vi "Func-엑셀 데이터를 그래프로 출력.vi"() -> ()   [LabVIEW 2015] (continued)
2.92\t19.328\n4.167\t2.85\t19.245\n4.083\t2.77\t19.179\n4\t2.68\t19.098\n3.917\t2.61\t19.025\n3.833\t2.53\t18.952\n3.75\t2.46\t18.87\n3.667\t2.38\t18.793\n3.583\t2.29\t18.723\n3.5\t2.22\t18.654\n3.417\t2.11\t18.582\n3.333\t2.03\t18.503\n3.25\t1.96\t18.435\n3.3\t1.89\t18.371\n3.3\t1.89\t18.367\n3.3\t1.88\t18.361\n3.3\t1.87\t18.354\n3.3\t1.86\t18.349\n3.3\t1.85\t18.337\n3.3\t1.85\t18.327\n3.3\t1.85\t18.316\n3.3\t1.84\t18.306\n3.3\t1.83\t18.299\n3.3\t1.83\t18.291\n3.3\t1.82\t18.284\n3.3\t1.81\t18.278\n3.3\t1.8\t18.274\n3.3\t1.79\t18.265\n3.3\t1.77\t18.259\n3.3\t1.77\t18.254\n3.3\t1.77\t18.244\n3.3\t1.75\t18.235\n3.3\t1.76\t18.228\n3.3\t1.74\t18.222\n3.3\t1.74\t18.214\n3.3\t1.72\t18.208\n3.3\t1.72\t18.2\n3.3\t1.7\t18.195\n3.3\t1.7\t18.186\n3.3\t1.69\t18.171\n3.3\t1.69\t18.166\n3.3\t1.69\t18.153\n3.3\t1.69\t18.148\n3.3\t1.68\t18.142\n3.3\t1.66\t18.139\n3.3\t1.65\t18.134\n3.3\t1.64\t18.131\n3.3\t1.64\t18.121\n3.3\t1.64\t18.115\n3.3\t1.63\t18.108\n3.3\t1.62\t18.097\n3.3\t1.62\t18.088\n3.3\t1.61\t18.081\n3.3\t1.61\t18.074\n3.3\t1.6\t18.065\n3.3\t1.6\t18.056\n3.3\t1.6\t18.046\n3.3\t1.59\t18.039\n3.3\t1.58\t18.031\n3.3\t1.58\t18.023\n3.3\t1.57\t18.019\n3.3\t1.57\t18.013\n3.3\t1.56\t18.006\n3.3\t1.55\t17.999\n3.3\t1.54\t17.993\n3.3\t1.53\t17.982\n3.3\t1.52\t17.974\n3.3\t1.52\t17.968\n3.3\t1.52\t17.958\n3.3\t1.52\t17.952\n3.3\t1.52\t17.945\n3.3\t1.52\t17.937\n3.3\t1.52\t17.93\n3.3\t1.51\t17.927\n3.3\t1.51\t17.919\n3.3\t1.5\t17.912\n3.3\t1.49\t17.907\n3.3\t1.49\t17.897\n3.3\t1.49\t17.892\n3.3\t1.48\t17.877\n3.3\t1.47\t17.871\n3.3\t1.48\t17.868\n3.3\t1.47\t17.86\n3.3\t1.46\t17.852\n3.3\t1.45\t17.846\n3.3\t1.45\t17.838\n3.3\t1.44\t17.832\n3.3\t1.43\t17.823\n3.3\t1.43\t17.814\n3.3\t1.43\t17.806\n3.3\t1.43\t17.8\n3.3\t1.42\t17.793\n3.3\t1.42\t17.788\n3.3\t1.41\t17.781\n3.3\t1.4\t17.771\n3.3\t1.4\t17.763\n3.3\t1.4\t17.755\n3.3\t1.4\t17.747\n3.3\t1.4\t17.74\n3.3\t1.4\t17.732\n3.3\t1.4\t17.725\n3.3\t1.4\t17.719\n3.3\t1.41\t17.709\n3.3\t1.4\t17.698\n3.3\t1.4\t17.689\n3.3\t1.39\t17.68\n3.3\t1.4\t17.672\n3.3\t1.39\t17.672\n3.3\t1.39\t17.668\n3.3\t1.39\t17.661\n3.3\t1.38\t17.658\n3.3\t1.39\t17.655\n3.3\t1.39\t17.643\n3.3\t1.39\t17.633\n3.3\t1.39\t17.627\n3.3\t1.4\t17.614\n3.3\t1.39\t17.607\n3.3\t1.4\t17.6\n3.3\t1.4\t17.593\n3.3\t1.4\t17.586\n3.3\t1.39\t17.579\n3.3\t1.39\t17.573\n3.3\t1.39\t17.565\n3.3\t1.39\t17.56\n3.3\t1.39\t17.554\n3.3\t1.39\t17.549\n3.3\t1.39\t17.545\n3.3\t1.39\t17.541\n3.3\t1.39\t17.533\n3.3\t1.39\t17.523\n3.3\t1.39\t17.509\n3.3\t1.4\t17.501\n3.3\t1.4\t17.493\n3.3\t1.41\t17.479\n3.3\t1.41\t17.474\n3.3\t1.4\t17.47\n3.3\t1.4\t17.466\n3.3\t1.4\t17.461\n3.3\t1.39\t17.452\n3.3\t1.4\t17.442\n3.3\t1.41\t17.435\n3.3\t1.4\t17.426\n3.3\t1.4\t17.416\n3.3\t1.41\t17.406\n3.3\t1.41\t17.4\n3.3\t1.41\t17.391\n3.3\t1.43\t17.386\n3.3\t1.43\t17.38\n3.3\t1.43\t17.37\n3.3\t1.43\t17.364\n3.3\t1.43\t17.356\n3.3\t1.43\t17.35\n3.3\t1.43\t17.34\n3.3\t1.43\t17.332\n3.3\t1.43\t17.321\n3.3\t1.43\t17.31\n3.3\t1.43\t17.303\n3.3\t1.43\t17.296\n3.3\t1.44\t17.29\n3.3\t1.44\t17.282\n3.3\t1.45\t17.275\n3.3\t1.45\t17.272\n3.3\t1.45\t17.268\n3.3\t1.46\t17.258\n3.3\t1.45\t17.252\n3.3\t1.46\t17.248\n3.3\t1.45\t17.236\n3.3\t1.47\t17.231\n3.3\t1.47\t17.225\n3.3\t1.48\t17.215\n3.3\t1.48\t17.21\n3.3\t1.49\t17.204\n3.3\t1.49\t17.199\n3.3\t1.48\t17.193\n3.3\t1.48\t17.185\n3.3\t1.49\t17.175\n3.3\t1.49\t17.168\n3.3\t1.5\t17.159\n3.3\t1.5\t17.152\n3.3\t1.5\t17.143\n3.3\t1.5\t17.135\n3.3\t1.51\t17.13\n3.3\t1.52\t17.121\n3.3\t1.52\t17.118\n3.3\t1.52\t17.109\n3.3\t1.53\t17.104\n3.3\t1.53\t17.099\n3.3\t1.53\t17.089\n3.3\t1.53\t17.083\n3.3\t1.53\t17.075\n3.3\t1.53\t17.07\n3.3\t1.54\t17.059\n3.3\t1.55\t17.051\n3.3\t1.55\t17.043\n3.3\t1.56\t17.036\n3.3\t1.57\t17.03\n3.3\t1.57\t17.018\n3.3\t1.57\t17.013\n3.3\t1.58\t17.009\n3.3\t1.58\t16.999\n3.3\t1.59\t16.991\n3.3\t1.6\t16.981\n3.3\t1.6\t16.971\n3.3\t1.61\t16.965\n3.3\t1.62\t16.955\n3.3\t1.62\t16.95\n3.3\t1.62\t16.95\n3.3\t1.62\t16.946\n3.3\t1.63\t16.938\n3.3\t1.64\t16.932\n3.3\t1.64\t16.921\n3.3\t1.65\t16.913\n3.3\t1.66\t16.902\n3.3\t1.66\t16.893\n3.3\t1.66\t16.888\n3.3\t1.67\t16.88\n3.3\t1.68\t16.875\n3.3\t1.69\t16.87\n3.3\t1.69\t16.867\n3.3\t1.69\t16.86\n3.3\t1.69\t16.854\n3.3\t1.7\t16.851\n3.3\t1.71\t16.843\n3.3\t1.72\t16.836\n3.3\t1.73\t16.828\n3.3\t1.74\t16.817\n3.3\t1.75\t16.81\n3.3\t1.75\t16.8\n3.3\t1.75\t16.791\n3.3\t1.76\t16.782\n3.3\t1.76\t16.772\n3.3\t1.76\t16.763\n3.3\t1.77\t16.757\n3.3\t1.77\t16.753\n3.3\t1.78\t16.745\n3.3\t1.78\t16.737\n3.3\t1.79\t16.734\n3.3\t1.8\t16.729\n3.3\t1.81\t16.72\n3.3\t1.81\t16.711\n3.3\t1.82\t16.702\n3.3\t1.83\t16.698\n3.3\t1.83\t16.688\n3.3\t1.84\t16.677\n3.3\t1.85\t16.675\n3.3\t1.85\t16.672\n3.3\t1.85\t16.663\n3.3\t1.86\t16.657\n3.3\t1.86\t16.653\n3.3\t1.87\t16.646\n3.3\t1.88\t16.637\n3.3\t1.89\t16.63\n3.3\t1.9\t16.625\n3.3\t1.91\t16.62\n3.3\t1.91\t16.617\n3.3\t1.92\t16.608\n3.3\t1.93\t16.604\n3.3\t1.94\t16.597\n3.3\t1.94\t16.584\n3.3\t1.94\t16.574\n3.3\t1.95\t16.569\n3.3\t1.95\t16.562\n3.3\t1.95\t16.55\n3.3\t1.96\t16.543\n3.3\t1.97\t16.536\n3.3\t1.98\t16.532\n3.3\t1.99\t16.524\n3.3\t2\t16.511\n3.3\t2.01\t16.507\n3.3\t2.02\t16.502\n3.3\t2.02\t16.493\n3.3\t2.03\t16.491\n3.3\t2.03\t16.483\n3.3\t2.04\t16.482\n3.3\t2.05\t16.478\n3.3\t2.05\t16.475\n3.3\t2.06\t16.468\n3.3\t2.07\t16.46\n3.3\t2.07\t16.451\n3.3\t2.07\t16.441\n3.3\t2.08\t16.435\n3.3\t2.09\t16.424\n3.3\t2.09\t16.416\n3.3\t2.1\t16.41\n3.3\t2.1\t16.4\n3.3\t2.11\t16.392\n3.3\t2.11\t16.385\n3.3\t2.12\t16.38\n3.3\t2.13\t16.376\n3.3\t2.14\t16.369\n3.3\t2.14\t16.36\n3.3\t2.15\t16.357\n3.3\t2.16\t16.351\n3.3\t2.17\t16.343\n3.3\t2.17\t16.336\n3.3\t2.18\t16.333\n3.3\t2.19\t16.334\n3.3\t2.19\t16.327\n3.3\t2.19\t16.32\n3.3\t2.2\t16.307\n3.3\t2.21\t16.298\n3.3\t2.22\t16.287\n3.3\t2.23\t16.274\n3.3\t2.24\t16.27\n3.3\t2.25\t16.265\n3.3\t2.25\t16.263\n3.3\t2.25\t16.262\n3.3\t2.25\t16.257\n3.3\t2.26\t16.251\n3.3\t2.27\t16.244\n3.3\t2.27\t16.236\n3.3\t2.28\t16.225\n3.3\t2.29\t16.218\n3.3\t2.3\t16.212\n3.3\t2.3\t16.204\n3.3\t2.31\t16.196\n3.3\t2.31\t16.195\n3.3\t2.32\t16.186\n3.3\t2.32\t16.179\n3.3\t2.33\t16.176\n3.3\t2.34\t16.169\n3.3\t2.35\t16.164\n3.3\t2.36\t16.155\n3.3\t2.36\t16.15\n3.3\t2.36\t16.145\n3.3\t2.36\t16.136\n3.3\t2.37\t16.127\n3.3\t2.37\t16.12\n3.3\t2.38\t16.112\n3.3\t2.39\t16.102\n3.3\t2.39\t16.096\n3.3\t2.4\t16.092\n3.3\t2.4\t16.085\n3.3\t2.4\t16.079\n3.3\t2.41\t16.074\n3.3\t2.42\t16.066\n3.3\t2.43\t16.06\n3.3\t2.44\t16.054\n3.3\t2.44\t16.044\n3.3\t2.44\t16.041\n3.3\t2.45\t16.038\n3.3\t2.45\t16.028\n3.3\t2.45\t16.022\n3.3\t2.46\t16.014\n3.3\t2.47\t16.007\n3.3\t2.48\t15.999\n3.3\t2.49\t15.994\n3.3\t2.5\t15.99\n3.3\t2.51\t15.984\n3.3\t2.51\t15.98\n3.3\t2.51\t15.973\n3.3\t2.52\t15.966\n3.3\t2.52\t15.96\n3.3\t2.52\t15.95\n3.3\t2.52\t15.945\n3.3\t2.52\t15.939\n3.3\t2.53\t15.93\n3.3\t2.53\t15.926\n3.3\t2.55\t15.92\n3.3\t2.55\t15.917\n3.3\t2.57\t15.909\n3.3\t2.57\t15.897\n3.3\t2.58\t15.894\n3.3\t2.58\t15.891\n3.3\t2.59\t15.884\n3.3\t2.6\t15.874\n3.3\t2.6\t15.871\n3.3\t2.61\t15.866\n3.3\t2.61\t15.859\n3.3\t2.61\t15.852\n3.3\t2.62\t15.848\n3.3\t2.63\t15.844\n3.3\t2.63\t15.841\n3.3\t2.63\t15.834\n3.3\t2.64\t15.831\n3.3\t2.65\t15.822\n3.3\t2.66\t15.812\n3.3\t2.66\t15.806\n3.3\t2.68\t15.799\n3.3\t2.68\t15.793\n3.3\t2.69\t15.786\n3.3\t2.69\t15.782\n3.3\t2.69\t15.774\n3.3\t2.69\t15.771\n3.3\t2.69\t15.762\n3.3\t2.69\t15.754\n3.3\t2.7\t15.748\n3.3\t2.71\t15.74\n3.3\t2.72\t15.732\n3.3\t2.73\t15.724\n3.3\t2.74\t15.721\n3.3\t2.74\t15.714\n3.3\t2.74\t15.709\n3.3\t2.75\t15.71\n3.3\t2.76\t15.703\n3.3\t2.77\t15.701\n3.3\t2.78\t15.697\n3.3\t2.78\t15.689\n3.3\t2.79\t15.684\n3.3\t2.79\t15.676\n3.3\t2.79\t15.666\n3.3\t2.8\t15.66\n3.3\t2.81\t15.652\n3.3\t2.82\t15.644\n3.3\t2.83\t15.637\n3.3\t2.84\t15.63\n3.3\t2.84\t15.624\n3.3\t2.84\t15.617\n3.3\t2.84\t15.614\n3.3\t2.84\t15.605\n3.3\t2.85\t15.603\n3.3\t2.86\t15.599\n3.3\t2.87\t15.592\n3.3\t2.87\t15.588\n3.3\t2.88\t15.582\n3.3\t2.88\t15.579\n3.3\t2.88\t15.572\n3.3\t2.88\t15.566\n3.3\t2.89\t15.563\n3.3\t2.89\t15.557\n3.3\t2.9\t15.552\n3.3\t2.91\t15.543\n3.3\t2.93\t15.536\n3.3\t2.92\t15.533\n3.3\t2.93\t15.523\n3.3\t2.93\t15.52\n3.3\t2.93\t15.514\n3.3\t2.93\t15.509\n3.3\t2.94\t15.507\n3.3\t2.94\t15.503\n3.3\t2.95\t15.497\n3.3\t2.95\t15.493\n3.3\t2.96\t15.488\n3.3\t2.97\t15.481\n3.3\t2.98\t15.473\n3.3\t2.98\t15.464\n3.3\t2.98\t15.455\n3.3\t2.99\t15.448\n3.3\t2.99\t15.447\n3.3\t2.99\t15.441\n3.3\t3\t15.435\n3.3\t3.01\t15.43\n3.3\t3.01\t15.425\n3.3\t3.01\t15.421\n3.3\t3.02\t15.414\n3.3\t3.02\t15.407\n3.3\t3.02\t15.404\n3.3\t3.02\t15.395\n3.3\t3.03\t15.391\n3.3\t3.03\t15.389\n3.3\t3.03\t15.382\n3.3\t3.03\t15.378\n3.3\t3.04\t15.373\n3.3\t3.04\t15.369\n3.3\t3.05\t15.363\n3.3\t3.05\t15.354\n3.3\t3.05\t15.346\n3.3\t3.05\t15.337\n3.3\t3.06\t15.335\n3.3\t3.07\t15.329\n3.3\t3.07\t15.328\n3.3\t3.08\t15.325\n3.3\t3.08\t15.319\n3.3\t3.08\t15.314\n3.3\t3.09\t15.307\n3.3\t3.09\t15.299\n3.3\t3.1\t15.291\n3.3\t3.1\t15.286\n3.3\t3.11\t15.283\n3.3\t3.11\t15.278\n3.3\t3.11\t15.272\n3.3\t3.11\t15.267\n3.3\t3.11\t15.264\n3.3\t3.11\t15.26\n3.3\t3.11\t15.252\n3.3\t3.11\t15.248\n3.3\t3.12\t15.248\n3.3\t3.13\t15.238\n3.3\t3.13\t15.232\n3.3\t3.13\t15.224\n3.3\t3.13\t15.216\n3.3\t3.14\t15.212\n3.3\t3.14\t15.208\n3.3\t3.14\t15.204\n3.3\t3.15\t15.199\n3.3\t3.15\t15.198\n3.3\t3.16\t15.195\n3.3\t3.16\t15.19\n3.3\t3.17\t15.187\n3.3\t3.17\t15.18\n3.3\t3.18\t15.175\n3.3\t3.18\t15.168\n3.3\t3.19\t15.163\n3.3\t3.19\t15.154\n3.3\t3.19\t15.146\n3.3\t3.19\t15.145\n3.3\t3.19\t15.142\n3.3\t3.19\t15.139\n3.3\t3.2\t15.131\n3.3\t3.2\t15.128\n3.3\t3.2\t15.123\n3.3\t3.2\t15.115\n3.3\t3.2\t15.112\n3.3\t3.21\t15.107\n3.3\t3.22\t15.103\n3.3\t3.22\t15.102\n3.3\t3.22\t15.096\n3.3\t3.23\t15.091\n3.3\t3.23\t15.084\n3.3\t3.23\t15.077\n3.3\t3.24\t15.07\n3.3\t3.25\t15.066\n3.3\t3.25\t15.063\n3.3\t3.24\t15.055\n3.3\t3.24\t15.049\n3.3\t3.25\t15.048\n3.3\t3.25\t15.042\n3.3\t3.25\t15.037\n3.3\t3.26\t15.031\n3.3\t3.26\t15.03\n3.3\t3.25\t15.028\n3.3\t3.25\t15.025\n3.3\t3.25\t15.021\n3.3\t3.26\t15.02\n3.3\t3.27\t15.016\n3.3\t3.28\t15.006\n3.3\t3.3\t15.001\n3.3\t3.3\t14.996\n3.3\t3.3\t14.988\n3.3\t3.3\t14.981\n3.3\t3.3\t14.979\n3.3\t3.3\t14.974\n3.3\t3.3\t14.969\n3.3\t3.3\t14.964\n3.3\t3.3\t14.961\n3.3\t3.3\t14.959\n3.3\t3.3\t14.952\n3.3\t3.3\t14.95\n3.3\t3.3\t14.948\n3.3\t3.3\t14.946\n3.3\t3.3\t14.94\n3.3\t3.3\t14.933\n3.3\t3.3\t14.931\n3.3\t3.3\t14.925\n3.3\t3.3\t14.92\n3.3\t3.3\t14.912\n3.3\t3.3\t14.9\n3.3\t3.3\t14.895\n3.3\t3.3\t14.889\n3.3\t3.3\t14.88\n3.3\t3.3\t14.873\n3.3\t3.3\t14.867\n3.3\t3.3\t14.866\n3.3\t3.3\t14.864\n3.3\t3.3\t14.862\n3.3\t3.3\t14.855\n3.3\t3.3\t14.855\n3.3\t3.3\t14.855\n3.3\t3.3\t14.848\n3.3\t3.3\t14.843\n3.3\t3.3\t14.84\n3.3\t3.3\t14.837\n3.3\t3.3\t14.836\n3.3\t3.3\t14.833\n3.3\t3.3\t14.83\n3.3\t3.3\t14.827\n3.3\t3.3\t14.823\n3.3\t3.3\t14.817\n3.3\t3.3\t14.813\n3.3\t3.31\t14.81\n3.3\t3.31\t14.805\n3.3\t3.31\t14.8\n3.3\t3.31\t14.798\n3.3\t3.31\t14.79\n3.3\t3.31\t14.787\n3.3\t3.31\t14.782\n3.3\t3.31\t14.778\n3.3\t3.31\t14.777\n3.3\t3.31\t14.77\n3.3\t3.31\t14.765\n3.3\t3.31\t14.758\n3.3\t3.31\t14.752\n3.3\t3.31\t14.743\n3.3\t3.31\t14.736\n3.3\t3.31\t14.734\n3.3\t3.31\t14.733\n3.3\t3.31\t14.727\n3.3\t3.31\t14.721\n3.3\t3.31\t14.715\n3.3\t3.31\t14.71\n3.3\t3.31\t14.708\n3.3\t3.31\t14.701\n3.3\t3.31\t14.698\n3.3\t3.31\t14.7\n3.3\t3.31\t14.7\n3.3\t3.31\t14.696\n3.3\t3.31\t14.691\n3.3\t3.31\t14.686\n3.3\t3.31\t14.684\n3.3\t3.31\t14.679\n3.3\t3.31\t14.673\n3.3\t3.31\t14.671\n3.3\t3.31\t14.667\n3.3\t3.31\t14.663\n3.3\t3.31\t14.659\n3.3\t3.31\t14.658\n3.3\t3.32\t14.653\n3.3\t3.32\t14.648\n3.3\t3.32\t14.644\n3.3\t3.32\t14.638\n3.3\t3.32\t14.63\n3.3\t3.32\t14.624\n3.3\t3.32\t14.62\n3.3\t3.32\t14.618\n3.3\t3.32\t14.616\n3.3\t3.32\t14.613\n3.3\t3.32\t14.609\n3.3\t3.32\t14.608\n3.3\t3.32\t14.603\n3.3\t3.32\t14.596\n3.3\t3.32\t14.591\n3.3\t3.32\t14.586\n3.3\t3.32\t14.585\n3.3\t3.32\t14.577\n3.3\t3.32\t14.575\n3.3\t3.32\t14.575\n3.3\t3.32\t14.567\n3.3\t3.32\t14.566\n3.3\t3.32\t14.561\n3.3\t3.32\t14.557\n3.3\t3.32\t14.55\n3.3\t3.32\t14.549\n3.3\t3.32\t14.55\n3.3\t3.32\t14.547\n3.3\t3.32\t14.546\n3.3\t3.32\t14.543\n3.3\t3.32\t14.541\n3.3\t3.32\t14.535\n3.3\t3.32\t14.526\n3.3\t3.32\t14.521\n3.3\t3.32\t14.513\n3.3\t3.32\t14.512\n3.3\t3.32\t14.511\n3.3\t3.32\t14.507\n3.3\t3.32\t14.507\n3.3\t3.32\t14.504\n3.3\t3.32\t14.505\n3.3\t3.32\t14.5\n3.3\t3.32\t14.496\n3.3\t3.32\t14.495\n3.3\t3.32\t14.491\n3.3\t3.32\t14.489\n3.3\t3.32\t14.486\n3.3\t3.32\t14.479\n3.3\t3.32\t14.477\n3.3\t3.32\t14.47\n3.3\t3.32\t14.467\n3.3\t3.32\t14.462\n3.3\t3.32\t14.457\n3.3\t3.32\t14.454\n3.3\t3.32\t14.449\n3.3\t3.32\t14.448\n3.3\t3.32\t14.44\n3.3\t3.32\t14.439\n3.3\t3.32\t14.435\n3.3\t3.32\t14.426\n3.3\t3.32\t14.421\n3.3\t3.32\t14.418\n3.3\t3.32\t14.412\n3.3\t3.32\t14.407\n3.3\t3.32\t14.407\n3.3\t3.32\t14.408\n3.3\t3.32\t14.41\n3.3\t3.32\t14.407\n3.3\t3.32\t14.407\n3.3\t3.32\t14.404\n3.3\t3.32\t14.396\n3.3\t3.32\t14.388\n3.3\t3.32\t14.387\n3.3\t3.32\t14.387\n3.3\t3.32\t14.383\n3.3\t3.32\t14.381\n3.3\t3.32\t14.382\n3.3\t3.32\t14.377\n3.3\t3.32\t14.367\n3.3\t3.32\t14.359\n3.3\t3.32\t14.349\n3.3\t3.32\t14.345\n3.3\t3.33\t14.343\n3.3\t3.32\t14.342\n3.3\t3.33\t14.34\n3.3\t3.33\t14.336\n3.3\t3.33\t14.332\n3.3\t3.32\t14.332\n3.3\t3.32\t14.329\n3.3\t3.32\t14.322\n3.3\t3.32\t14.319\n3.3\t3.32\t14.32\n3.3\t3.33\t14.318\n3.3\t3.33\t14.313\n3.3\t3.33\t14.311\n3.3\t3.33\t14.311\n3.3\t3.33\t14.31\n3.3\t3.33\t14.306\n3.3\t3.32\t14.303\n3.3\t3.32\t14.301\n3.3\t3.32\t14.295\n3.3\t3.32\t14.291\n3.3\t3.33\t14.288\n3.3\t3.33\t14.284\n3.3\t3.33\t14.28\n3.3\t3.33\t14.275\n3.3\t3.33\t14.272\n3.3\t3.33\t14.268\n3.3\t3.33\t14.264\n3.3\t3.33\t14.264\n3.3\t3.33\t14.259\n3.3\t3.33\t14.257\n3.3\t3.33\t14.255\n3.3\t3.33\t14.252\n3.3\t3.33\t14.246\n3.3\t3.33\t14.241\n3.3\t3.33\t14.237\n3.3\t3.33\t14.233\n3.3\t3.33\t14.231\n3.3\t3.32\t14.223\n3.3\t3.32\t14.225\n3.3\t3.32\t14.223\n3.3\t3.32\t14.222\n3.3\t3.32\t14.22\n3.3\t3.32\t14.216\n3.3\t3.32\t14.216\n3.3\t3.33\t14.212\n3.3\t3.33\t14.208\n3.3\t3.33\t14.203\n3.3\t3.33\t14.196\n3.3\t3.32\t14.193\n3.3\t3.32\t14.191\n3.3\t3.32\t14.188\n3.3\t3.32\t14.183\n3.3\t3.32\t14.181\n3.3\t3.32\t14.182\n3.3\t3.32\t14.184\n3.3\t3.32\t14.181\n3.3\t3.32\t14.176\n3.3\t3.32\t14.179\n3.3\t3.32\t14.175\n3.3\t3.32\t14.173\n3.3\t3.32\t14.166\n3.3\t3.32\t14.159\n3.3\t3.32\t14.157\n3.3\t3.32\t14.153\n3.3\t3.32\t14.154\n3.3\t3.32\t14.152\n3.3\t3.32\t14.15\n3.3\t3.32\t14.15\n3.3\t3.32\t14.148\n3.3\t3.32\t14.145\n3.3\t3.32\t14.134\n3.3\t3.32\t14.131\n3.3\t3.32\t14.128\n3.3\t3.32\t14.123\n3.3\t3.32\t14.119\n3.3\t3.32\t14.118\n3.3\t3.32\t14.116\n3.3\t3.32\t14.11\n3.3\t3.32\t14.11\n3.3\t3.32\t14.104\n3.3\t3.32\t14.104\n3.3\t3.32\t14.098\n3.3\t3.32\t14.095\n3.3\t3.32\t14.099\n3.3\t3.32\t14.094\n3.3\t3.32\t14.091\n3.3\t3.32\t14.088\n3.3\t3.32\t14.087\n3.3\t3.32\t14.086\n3.3\t3.32\t14.079\n3.3\t3.32\t14.075\n3.3\t3.32\t14.07\n3.3\t3.32\t14.066\n3.3\t3.32\t14.064\n3.3\t3.32\t14.061\n3.3\t3.32\t14.059\n3.3\t3.32\t14.057\n3.3\t3.32\t14.056\n3.3\t3.32\t14.054\n3.3\t3.32\t14.05\n3.3\t3.32\t14.048\n3.3\t3.32\t14.044\n3.3\t3.32\t14.044\n3.3\t3.32\t14.039\n3.3\t3.32\t14.036\n3.3\t3.32\t14.031\n3.3\t3.32\t14.025\n3.3\t3.32\t14.025\n3.3\t3.32\t14.024\n3.3\t3.32\t14.019\n3.3\t3.32\t14.017\n3.3\t3.32\t14.02\n3.3\t3.32\t14.016\n3.3\t3.32\t14.013\n3.3\t3.32\t14.009\n3.3\t3.32\t14.01\n3.3\t3.32\t14.008\n3.3\t3.32\t14.004\n3.3\t3.32\t13.998\n3.3\t3.32\t13.994\n3.3\t3.32\t13.994\n3.3\t3.32\t13.986\n3.3\t3.32\t13.985\n3.3\t3.32\t13.979\n3.3\t3.32\t13.979\n3.3\t3.32\t13.979\n3.3\t3.32\t13.976\n3.3\t3.32\t13.973\n3.3\t3.32\t13.971\n3.3\t3.31\t13.969\n3.3\t3.31\t13.966\n3.3\t3.31\t13.962\n3.3\t3.31\t13.96\n3.3\t3.31\t13.959\n3.3\t3.31\t13.954\n3.3\t3.31\t13.951\n3.3\t3.31\t13.944\n3.3\t3.31\t13.943\n3.3\t3.31\t13.941\n3.3\t3.31\t13.939\n3.3\t3.31\t13.939\n3.3\t3.31\t13.939\n3.3\t3.31\t13.94\n3.3\t3.31\t13.936\n3.3\t3.31\t13.932\n3.3\t3.31\t13.927\n3.3\t3.31\t13.925\n3.3\t3.31\t13.92\n3.3\t3.31\t13.918\n3.3\t3.31\t13.914\n3.3\t3.31\t13.913\n3.3\t3.31\t13.91\n3.3\t3.31\t13.908\n3.3\t3.31\t13.905\n3.3\t3.31\t13.9\n3.3\t3.31\t13.898\n3.3\t3.31\t13.898\n3.3\t3.31\t13.893\n3.3\t3.31\t13.889\n3.3\t3.31\t13.889\n3.3\t3.31\t13.887\n3.3\t3.31\t13.886\n3.3\t3.31\t13.88\n3.3\t3.31\t13.878\n3.3\t3.31\t13.877\n3.3\t3.31\t13.875\n3.3\t3.31\t13.876\n3.3\t3.31\t13.871\n3.3\t3.31\t13.871\n3.3\t3.31\t13.869\n3.3\t3.31\t13.866\n3.3\t3.31\t13.865\n3.3\t3.31\t13.859\n3.3\t3.31\t13.863\n3.3\t3.31\t13.86\n3.3\t3.31\t13.858\n3.3\t3.31\t13.859\n3.3\t3.31\t13.854\n3.3\t3.31\t13.852\n3.3\t3.31\t13.845\n3.3\t3.31\t13.837\n3.3\t3.31\t13.837\n3.3\t3.31\t13.834\n3.3\t3.31\t13.831\n3.3\t3.31\t13.831\n3.3\t3.31\t13.831\n3.3\t3.31\t13.832\n3.3\t3.31\t13.827\n3.3\t3.31\t13.826\n3.3\t3.31\t13.82\n3.3\t3.31\t13.816\n3.3\t3.31\t13.813\n3.3\t3.31\t13.814\n3.3\t3.31\t13.812\n3.3\t3.31\t13.806\n3.3\t3.31\t13.807\n3.3\t3.31\t13.806\n3.3\t3.31\t13.804\n3.3\t3.31\t13.8\n3.3\t3.31\t13.799\n3.3\t3.31\t13.798\n3.3\t3.31\t13.796\n3.3\t3.3\t13.794\n3.3\t3.3\t13.795\n3.3\t3.3\t13.79\n3.3\t3.3\t13.787\n3.3\t3.31\t13.788\n3.3\t3.31\t13.788\n3.3\t3.31\t13.782\n3.3\t3.31\t13.778\n3.3\t3.31\t13.776\n3.3\t3.31\t13.773\n3.3\t3.31\t13.771\n3.3\t3.31\t13.769\n3.3\t3.31\t13.769\n3.3\t3.31\t13.767\n3.3\t3.31\t13.765\n3.3\t3.31\t13.764\n3.3\t3.31\t13.761\n3.3\t3.31\t13.755\n3.3\t3.31\t13.746\n3.3\t3.31\t13.745\n3.3\t3.31\t13.745\n3.3\t3.31\t13.739\n3.3\t3.31\t13.738\n3.3\t3.31\t13.74\n3.3\t3.31\t13.743\n3.3\t3.31\t13.739\n3.3\t3.31\t13.734\n3.3\t3.3\t13.732\n3.3\t3.3\t13.728\n3.3\t3.3\t13.726\n3.3\t3.3\t13.723\n3.3\t3.3\t13.723\n3.3\t3.3\t13.721\n3.3\t3.3\t13.714\n3.3\t3.3\t13.711\n3.3\t3.3\t13.709\n3.3\t3.3\t13.707\n3.3\t3.3\t13.705\n3.3\t3.3\t13.705\n3.3\t3.3\t13.706\n3.3\t3.3\t13.707\n3.3\t3.3\t13.702\n3.3\t3.3\t13.696\n3.3\t3.3\t13.693\n3.3\t3.3\t13.69\n3.3\t3.3\t13.687\n3.3\t3.3\t13.686\n3.3\t3.3\t13.687\n3.3\t3.3\t13.687\n3.3\t3.3\t13.686\n3.3\t3.3\t13.68\n3.3\t3.3\t13.678\n3.3\t3.3\t13.676\n3.3\t3.3\t13.673\n3.3\t3.3\t13.666\n3.3\t3.3\t13.666\n3.3\t3.3\t13.667\n3.3\t3.3\t13.666\n3.3\t3.3\t13.661\n3.3\t3.3\t13.657\n3.3\t3.3\t13.655\n3.3\t3.3\t13.655\n3.3\t3.3\t13.648\n3.3\t3.3\t13.645\n3.3\t3.3\t13.642\n3.3\t3.3\t13.641\n3.3\t3.3\t13.641\n3.3\t3.3\t13.641\n3.3\t3.3\t13.644\n3.3\t3.3\t13.641\n3.3\t3.3\t13.644\n3.3\t3.3\t13.639\n3.3\t3.3\t13.637\n3.3\t3.3\t13.635\n3.3\t3.3\t13.632\n3.3\t3.3\t13.63\n3.3\t3.3\t13.628\n3.3\t3.3\t13.628\n3.3\t3.3\t13.625\n3.3\t3.3\t13.623\n3.3\t3.3\t13.618\n3.3\t3.3\t13.618\n3.3\t3.3\t13.617\n3.3\t3.3\t13.612\n3.3\t3.3\t13.61\n3.3\t3.3\t13.608\n3.3\t3.3\t13.605\n3.3\t3.3\t13.603\n3.3\t3.3\t13.6\n3.3\t3.3\t13.599\n3.3\t3.3\t13.6\n3.3\t3.3\t13.598\n3.3\t3.3\t13.594\n3.3\t3.3\t13.591\n3.3\t3.3\t13.591\n3.3\t3.3\t13.589\n3.3\t3.3\t13.585\n3.3\t3.3\t13.582\n3.3\t3.3\t13.586\n3.3\t3.3\t13.586\n3.3\t3.3\t13.581\n3.3\t3.3\t13.576\n3.3\t3.3\t13.572\n3.3\t3.3\t13.57\n3.3\t3.3\t13.566\n3.3\t3.3\t13.561\n3.3\t3.3\t13.558\n3.3\t3.3\t13.557\n3.3\t3.3\t13.556\n3.3\t3.3\t13.557\n3.3\t3.3\t13.553\n3.3\t3.3\t13.552\n3.3\t3.3\t13.553\n3.3\t3.3\t13.549\n3.3\t3.3\t13.549\n3.3\t3.3\t13.548\n3.3\t3.3\t13.546\n3.3\t3.3\t13.545\n3.3\t3.3\t13.545\n3.3\t3.3\t13.545\n3.3\t3.3\t13.544\n3.3\t3.3\t13.539\n3.3\t3.3\t13.538\n3.3\t3.3\t13.534\n3.3\t3.3\t13.53\n3.3\t3.3\t13.529\n3.3\t3.3\t13.527\n3.3\t3.3\t13.526\n3.3\t3.3\t13.525\n3.3\t3.3\t13.527\n3.3\t3.3\t13.523\n3.3\t3.3\t13.517\n3.3\t3.3\t13.514\n3.3\t3.3\t13.512\n3.3\t3.3\t13.512\n3.3\t3.3\t13.508\n3.3\t3.3\t13.509\n3.3\t3.3\t13.51\n3.3\t3.3\t13.507\n3.3\t3.3\t13.504\n3.3\t3.3\t13.495\n3.3\t3.3\t13.493\n3.3\t3.3\t13.493\n3.3\t3.3\t13.488\n3.3\t3.3\t13.486\n3.3\t3.3\t13.486\n3.3\t3.3\t13.486\n3.3\t3.3\t13.486\n3.3\t3.3\t13.484\n3.3\t3.3\t13.484\n3.3\t3.3\t13.486\n3.3\t3.3\t13.484\n3.3\t3.3\t13.482\n3.3\t3.3\t13.483\n3.3\t3.3\t13.478\n3.3\t3.3\t13.475\n3.3\t3.3\t13.473\n3.3\t3.3\t13.471\n3.3\t3.3\t13.469\n3.3\t3.3\t13.468\n3.3\t3.3\t13.466\n3.3\t3.3\t13.465\n3.3\t3.3\t13.464\n3.3\t3.3\t13.466\n3.3\t3.3\t13.462\n3.3\t3.3\t13.457\n3.3\t3.3\t13.459\n3.3\t3.3\t13.456\n3.3\t3.3\t13.451\n3.3\t3.3\t13.447\n3.3\t3.3\t13.446\n3.3\t3.3\t13.444\n3.3\t3.3\t13.436\n3.3\t3.3\t13.432\n3.3\t3.3\t13.432\n3.3\t3.3\t13.432\n3.3\t3.3\t13.43\n3.3\t3.3\t13.433\n3.3\t3.3\t13.436\n3.3\t3.3\t13.436\n3.3\t3.3\t13.432\n3.3\t3.3\t13.43\n3.3\t3.3\t13.429\n
